vi "Data Replay DBLs to Waveform.vi"(8 "cycle range":u16=720, 9 "display two rotations? (F)":bool, 10 "Position reference":T1, 11 "Data":dbl[](array[numeric])) -> (3 "waveform":waveform(dbl))   [LabVIEW 2020, in "Engine Simulation Toolkit System Explorer.lvlib"]
uses:
  Engine Simulation Toolkit System Explorer.lvlib
  Position Reference.ctl
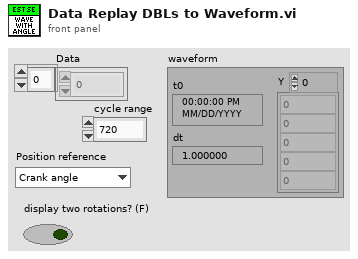
[diagram p1: front panel]
types:
  T1 = typedef "Engine Simulation Toolkit System Explorer.lvlib/Position Reference.ctl" = enum16{"Crank angle", "Cycle angle"}
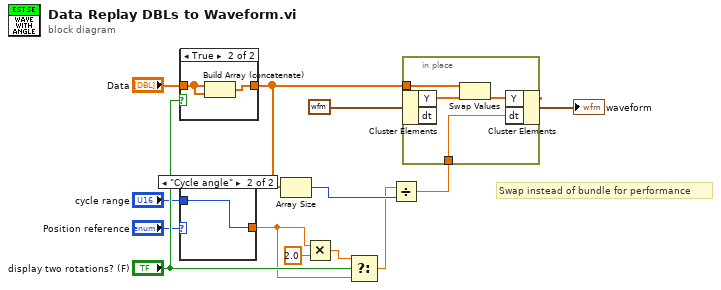
[diagram p0: block diagram]
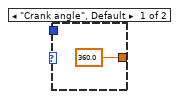
[diagram p2: hidden frame]
diagram:
  # "Swap instead of bundle for performance"
  n1 = case shown="True" "display two rotations? (F)" {
    tunnel: [w14 w16] -> w6
    tunnel: "Data" -> [w14 w15]
    frame False {
    }
    frame True {
      n2 = Build Array (concatenate)(w15, w15) -> (w16:dbl[])
    }
  }
  n3 = case shown="\"Cycle angle\"" "Position reference" {
    tunnel: [360.0 ("f") w18] -> w2
    tunnel: "cycle range" -> [_ w18]
    frame "Crank angle", Default {
    }
    frame "Cycle angle" {
    }
  }
  n4 = Array Size(array=w6) -> (size(s)=w11:i32)
  n5 = Multiply(x=w2, y=2.0) -> (x*y=w9:dbl)
  n6 = Select(t=w9, s="display two rotations? (F)", f=w2) -> (s? t:f=w7:dbl)
  n7 = Divide(x=w7, y=w11) -> (x/y=w12:dbl)
  n8 = in-place {
    in-place-border: w6 -> [w21]
    in-place-border: w12 -> [w19]
    n9 = in-place-cluster #1(waveform(dbl) {"t0"=timestamp(0 s since 1904-01-01), "dt"=1.0, "Y"=[]} ("waveform")) -> ("Y"=w22:dbl[])  [unwired: 1 out]
    n10 = Swap Values(12:w21, 14:w22) -> (3:w20:dbl[])  [unwired: 1 in, 1 out]
    n11 = in-place-cluster #1("Y"=w20, "dt"=w19) -> (→"waveform":waveform(dbl))
  }
